vi "Write data.vi"(8 "error in (no error)":errorcluster, 10 "data":T15={"Stop"=FALSE, "dataType"=enum."interferogram", "spectrometerIdx"=0, "buffer size interferogram"=0, "interferogram"={"new"=FALSE, "plot_x_ min"=0.0, "plot_x_max"=0.0, "plot_y_min"=0.0, "plot_y_max"=0.0, "Graph Intrfrgrm"=refnum, "timeStamp"=0, "signal (%)"=0.0, "traces"=[], "traces idx last"=0}, "spectrum"={"new"=FALSE, "plot_x_min"=0.0, "plot_x_max"=0.0, "plot_unit_x"=enum."wavenr/cm", "plot_unit_y"=enum."ADC counts", "plot_y_min"=0.0, "plot_y_max"=0.0, "Graph Spectrum"=refnum, "timeStamp"=0, "X_VAL_OPTIONS"=enum."MIN_MAX", "traces"=[], "traces idx last"=0}, "Thorlabs_OSA_64.lvclass:queue_action.ctlqueue ref"=refnum, "action"=enum."none", "plot zoom step"=0.0, "buffer semaphore"=refnum, "acq stopped"=FALSE, "dataType active"=enum."interferogram", "temperature (degr C)"=0.0, "pressure (hPa)"=0.0, "rel humidity (%)"=0.0, "settings"={"resolution"=0, "sensitivity"=0, "Average"=FALSE, "average nr"=1, "apodisation"=enum."NONE", "acq delay (ms)"=500, "airMesure"=enum."TEMPERATURE", "wmtr on"=FALSE, "intfgrm_smooth_width"=0, "intfgrm_smooth_nrOfPasses"=0, "intfgrm_smooth"=enum."NONE", "phaseCorrection"=enum."NONE", "zeroFill"=0, "spectr_smooth"=enum."NONE", "spectr_smooth_width"=0, "spectr_smooth_nrOfPasses"=0, "resolution (/cm)"=0.0, "REF wavelength, (nm)"=0.0, "gain_idx"=0, "gainAuto"=FALSE, "gain_relative"=0.0, "PD sensitivity mode"=enum."cool: better sensitivity/noise floor", "PD senseMode implemented"=FALSE, "SensorTemperature implemented"=FALSE, "SensorPressure implemented"=FALSE, "SensorHumidity implemented"=FALSE}, "peaks position"=[], "peaks width"=[], "peaks height"=[], "peaks max nr"=0, "peaks latest nr"=0, "peaks new"=FALSE, "power"=0.0, "power new"=FALSE, "path"="", "wavelength (WNr)"=0.0, "wavelength new"=FALSE, "buffer size spectrum"=0, "status"="", "VI reference"=refnum, "funcPointer"=0, "libraryPointer"=0, "singleAcquisition"=FALSE, "coherenceLength (cm)"=0.0, "coherenceLength new"=FALSE, "spectrometer model"="", "spectrometer serial nr"="", "peaks thld left"=[], "peaks thld right"=[], "coherenceLength error (cm)"=0.0, "ADC bits"=0, "peaks position centroid"=[], "peaks height centroid"=[], "OSA series"=enum."OSA200", "channel index spectrum"=0, "spectrometer rangeLow, (/cm)"=0.0, "spectrometer rangeHigh, (/cm)"=0.0, "channel index interferogram"=0} {"peaks height centroid" format="%.2f"; "peaks position centroid" format="%.2f"; "coherenceLength error (cm)" format="%.2f"; "peaks thld right" format="%.2f"; "peaks thld left" format="%.2f"; "coherenceLength (cm)" format="%.2f"; "wavelength (WNr)" format="%.2f"; "power" format="%.2f"; "peaks height" format="%.2f"; "peaks width" format="%.2f"; "peaks position" format="%.2f"; "settings"."REF wavelength, (nm)" format="%.2f"; "settings"."resolution (/cm)" format="%.2f"; "settings"."acq delay (ms)" step=200; "settings"."average nr" min=1 max=100 step=1; "settings"."sensitivity" items=["low", "low medium", "high medium", "high"]; "settings"."resolution" items=["low", "high"]; "rel humidity (%)" format="%.2f"; "pressure (hPa)" format="%.2f"; "temperature (degr C)" format="%.2f"; "plot zoom step" format="%.2f"; "spectrum"."plot_y_max" format="%.2f"; "spectrum"."plot_y_min" format="%.2f"; "spectrum"."plot_x_max" format="%.2f"; "spectrum"."plot_x_min" format="%.2f"; "interferogram"."plot_y_max" format="%.2f"; "interferogram"."plot_y_min" format="%.2f"; "interferogram"."plot_x_max" format="%.2f"; "interferogram"."plot_x_ min" format="%.2f"}, 11 "OSA_FTS in":refnum<class "OSA_FTS.lvclass">) -> (0 "error out":errorcluster, 3 "OSA_FTS out":refnum<class "OSA_FTS.lvclass">)   [LabVIEW 2010, in "OSA_FTS.lvclass"]
uses:
  OSA_FTS.lvclass
  typeDef/acq_dataType.ctl
  OSA.lvclass
  private/graph_intensity.ctl
  typeDef/spectrum_x_unit.ctl
  typeDef/y_unit.ctl
  typeDef/queue_action.ctl
  misc_examples/action_data.ctl
  typeDef/resolution.ctl
  typeDef/sensitivityMode.ctl
  typeDef/apodisation.ctl
  typeDef/airMeasure.ctl
  _misc/Thorlabs_FTS_misc.llb/interferogram_smoothing.ctl
  OSA20X_misc.lvlib
  typeDef/phaseCorrection.ctl
  _misc/Thorlabs_FTS_misc.llb/PDTemperatureMode.ctl
  typeDef/OSA_series.ctl
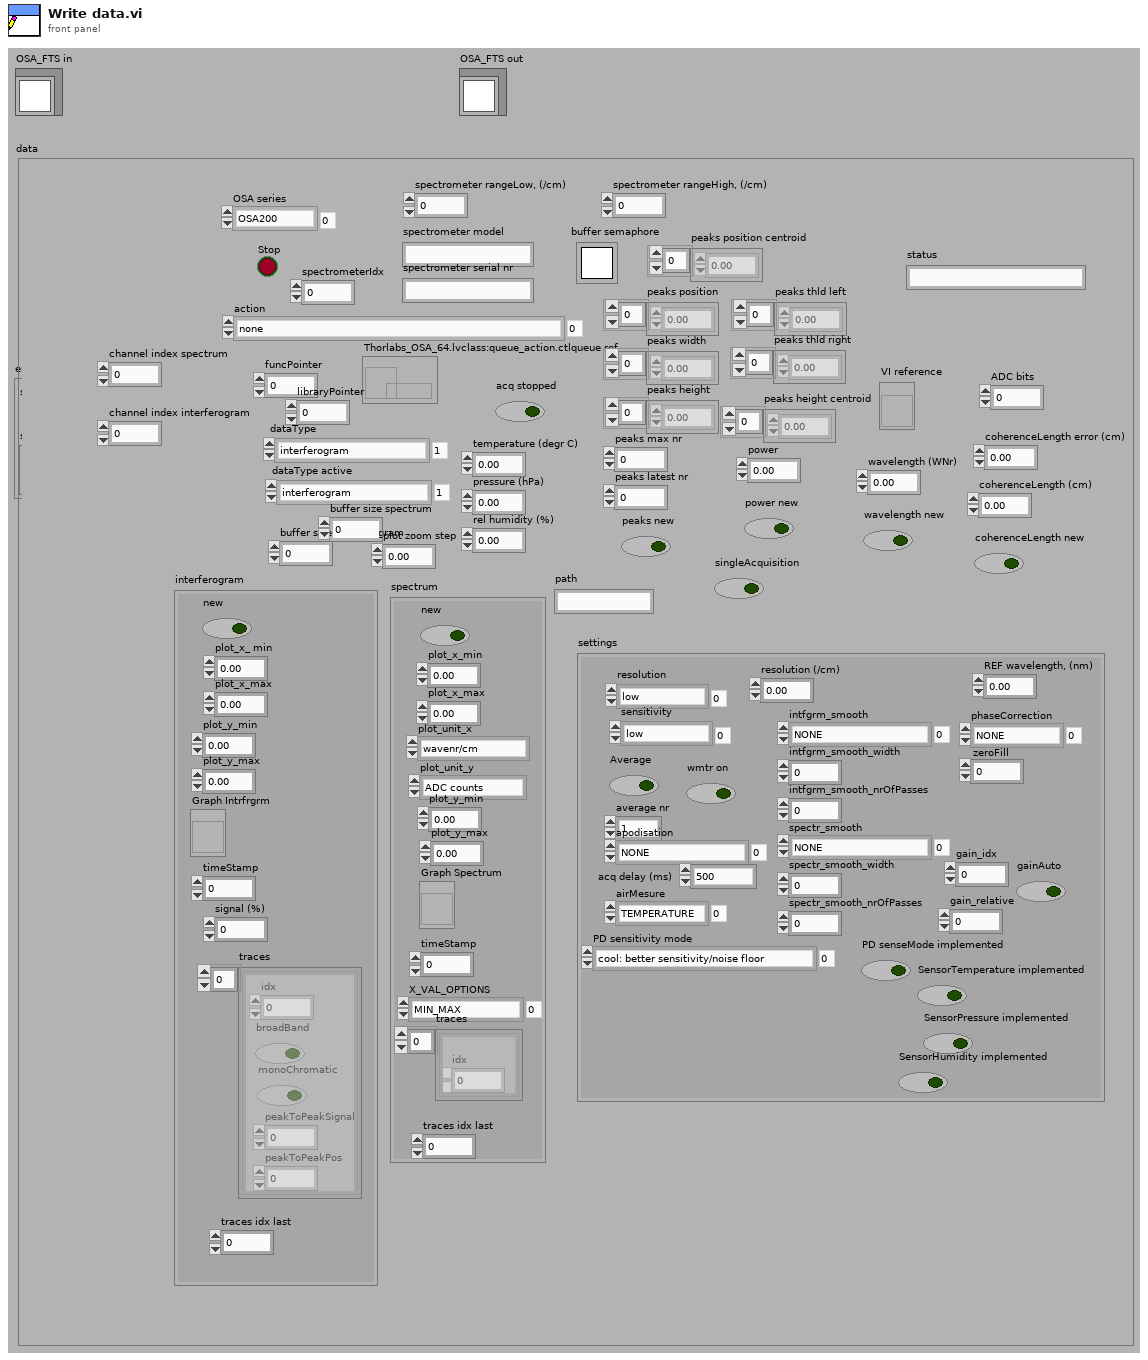
[diagram p1: front panel]
types:
  T1 = typedef "OSA.lvclass/acq_dataType.ctl" = enum16{"none", "interferogram", "spectrum"}
  T2 = typedef "OSA.lvclass/graph_intensity.ctl" = refnum<vi>
  T3 = typedef "OSA.lvclass/spectrum_x_unit.ctl" = enum16{"wavenr/cm", "THz", "eV", "nm_air", "nm_vac"}
  T4 = typedef "OSA.lvclass/y_unit.ctl" = enum16{"ADC counts", "dBm pwr absolute", "dBm pwr density", "mW pwr absolute", "mW pwr density"}
  T5 = typedef "OSA.lvclass/queue_action.ctl" = enum16{"none", "stop", "GUI_plotInterferogram", "GUI_plotSpectrum", "GUI_plotInterferogramRescale", "GUI_plotSpectrumRescale", "GUI_plotInterferogramReset", "GUI_plotSpectrumReset", "GUI_plotInterferogramAutoScaleY", "GUI_plotSpectrumAutoScaleY", "GUI_plotInterferogramZoomOut", "GUI_plotSpectrumZoomOut", "GUI_plotInterferogramPane", "GUI_plotSpectrumPane", "GUI_plotInterferogramZoomMouse", "GUI_plotSpectrumZoomMouse", "GUI_spectrumChannelType", "GUI_channel", "ENVIRONMENT temperature", "ENVIRONMENT pressure", "MODE_resolution set", "MODE_resolution get", "MODE_sensitivity set", "MODE_sensitivity get", "MODE_PDTemperature set", "MODE_PDTemperature get", "REBOOT/RESET firmware", "ACQASYNC_acquireSingleSpectrum", "ACQASYNC_continuous start", "ACQASYNC_continuous stop\n", "ACQASYNC_get last interferogram", "ACQASYNC_get last spectrum", "ACQASYNC_get last waveNr", "ACQOPT_interferogram smoothing set", "ACQOPT_interferogram smoothing get", "ACQOPT_spectrum smoothing set", "ACQOPT_spectrum smoothing get", "ACQOPT_apodisation type set", "ACQOPT_apodisation type get", "ACQOPT_phase correction type set", "ACQOPT_phase correction type get", "ACQOPT_acqIntervall_set", "ACQOPT_acqIntervall_get", "ACQOPT_average spectrum set", "ACQOPT_average spectrum get", "ACQOPT_rolling average set", "ACQOPT_rolling average get", "ACQOPT_zero fill factor set", "ACQOPT_zero fill factor get", "ACQOPT_cycle counting set", "ACQOPT_cycle counting get", "ACQOPT_air measure option set", "ACQOPT_air measure option get", "ACQOPT_gainLevel auto get", "ACQOPT_gainLevel auto set", "ACQOPT_gainLevel get", "ACQOPT_gainLevel set", "ACQOPT_offset set", "ACQOPT_attenuator_auto_set", "ACQOPT_attenuator_set", "ACQOPT_getAll", "INSTRUMENT_PROPERTY_range_WaveNr_min", "INSTRUMENT_PROPERTY_range_WaveNr_max", "INSTRUMENT_PROPERTY_reference_wavelength_cm^-1", "INSTRUMENT_PROPERTY_samplesPerRefPeriod", "INSTRUMENT_PROPERTY_resolution_waveNrPercm", "INSTRUMENT_PROPERTY_availableGainLevels", "INSTRUMENT_PROPERTY_status", "CONVERT", "ANALYSE_POWER", "ANALYSE_PEAKS", "ANALYSE_WAVELENGTH", "ANALYSE_SPECTRUM", "ANALYSE_INTERFEROGRAM", "ANALYSE_COHERENCE_LENGTH", "MATH", "MATH_power", "MATH_peaks", "FILE", "miscellaneous"}
  T6 = typedef "Semaphore RefNum" = refnum<k1>
  T7 = typedef "OSA.lvclass/resolution.ctl" = u16
  T8 = typedef "OSA.lvclass/sensitivityMode.ctl" = u16
  T9 = typedef "OSA.lvclass/apodisation.ctl" = enum16{"NONE", "NORTON_BEER_WEAK", "NORTON_BEER_MEDIUM", "NORTON_BEER_STRONG", "TRIANGULAR", "COSINE", "HANN", "HAMMING", "BLACKMANHARRIS3", "BLACKMANHARRIS4", "GAUSSIAN"}
  T10 = typedef "OSA.lvclass/airMeasure.ctl" = enum16{"TEMPERATURE", "PRESSURE"}
  T11 = typedef "OSA20X_misc.lvlib/interferogram_smoothing.ctl" = enum16{"NONE", "BINOMIAL", "SAVITSKY_GOLAY", "FOURIER", "MOVING_AVERAGE", "GAUSSIAN"}
  T12 = typedef "OSA.lvclass/phaseCorrection.ctl" = enum16{"NONE", "MERTZ", "FORMAN", "MERTZ_FILE", "FORMAN_FILE", "FUTURE COMP."}
  T13 = typedef "OSA20X_misc.lvlib/PDTemperatureMode.ctl" = enum16{"cool: better sensitivity/noise floor", "warm: extended wl range"}
  T14 = typedef "OSA.lvclass/OSA_series.ctl" = enum16{"OSA200", "OSA300", "UNKNOWN"}
  T15 = cluster{"Stop":bool, "dataType":T1, "spectrometerIdx":u16, "buffer size interferogram":i32, "interferogram":cluster{"new":bool, "plot_x_ min":sgl, "plot_x_max":sgl, "plot_y_min":sgl, "plot_y_max":sgl, "Graph Intrfrgrm":T2, "timeStamp":u32, "signal (%)":dbl, "traces":cluster{"idx":u32, "broadBand":bool, "monoChromatic":bool, "peakToPeakSignal":dbl, "peakToPeakPos":dbl}[], "traces idx last":i32}, "spectrum":cluster{"new":bool, "plot_x_min":sgl, "plot_x_max":sgl, "plot_unit_x":T3, "plot_unit_y":T4, "plot_y_min":sgl, "plot_y_max":sgl, "Graph Spectrum":T2, "timeStamp":u32, "X_VAL_OPTIONS":enum16{"MIN_MAX", "ARRAY"}, "traces":cluster{"idx":u32}[], "traces idx last":i32}, "Thorlabs_OSA_64.lvclass:queue_action.ctlqueue ref":refnum<queue>, "action":T5, "plot zoom step":dbl, "buffer semaphore":T6, "acq stopped":bool, "dataType active":T1, "temperature (degr C)":sgl, "pressure (hPa)":sgl, "rel humidity (%)":sgl, "settings":cluster{"resolution":T7, "sensitivity":T8, "Average":bool, "average nr":u32, "apodisation":T9, "acq delay (ms)":u32, "airMesure":T10, "wmtr on":bool, "intfgrm_smooth_width":u16, "intfgrm_smooth_nrOfPasses":u16, "intfgrm_smooth":T11, "phaseCorrection":T12, "zeroFill":u8, "spectr_smooth":T11, "spectr_smooth_width":u16, "spectr_smooth_nrOfPasses":u16, "resolution (/cm)":sgl, "REF wavelength, (nm)":dbl, "gain_idx":u16, "gainAuto":bool, "gain_relative":dbl, "PD sensitivity mode":T13, "PD senseMode implemented":bool, "SensorTemperature implemented":bool, "SensorPressure implemented":bool, "SensorHumidity implemented":bool}, "peaks position":sgl[], "peaks width":sgl[], "peaks height":sgl[], "peaks max nr":u32, "peaks latest nr":i32, "peaks new":bool, "power":dbl, "power new":bool, "path":string, "wavelength (WNr)":dbl, "wavelength new":bool, "buffer size spectrum":i32, "status":string, "VI reference":refnum<vi>, "funcPointer":u64, "libraryPointer":u64, "singleAcquisition":bool, "coherenceLength (cm)":dbl, "coherenceLength new":bool, "spectrometer model":string, "spectrometer serial nr":string, "peaks thld left":sgl[], "peaks thld right":sgl[], "coherenceLength error (cm)":dbl, "ADC bits":u16, "peaks position centroid":sgl[], "peaks height centroid":sgl[], "OSA series":T14, "channel index spectrum":u16, "spectrometer rangeLow, (/cm)":dbl, "spectrometer rangeHigh, (/cm)":dbl, "channel index interferogram":u16}
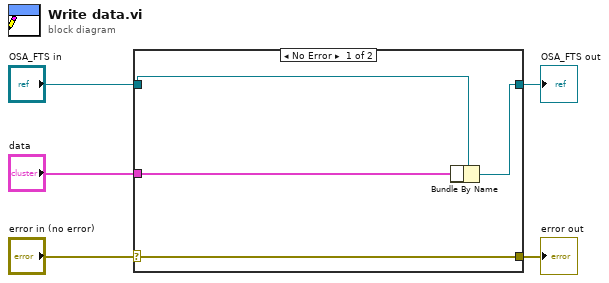
[diagram p0: block diagram]
diagram:
  n1 = case shown="No Error" "error in (no error)" {
    selector: "error in (no error)" -> [w9 w10]
    tunnel: [w9 w10] -> w4
    tunnel: [w7 w11] -> w2
    tunnel: "OSA_FTS in" -> [w8 w11]
    tunnel: "data" -> [w6 _]
    frame No Error {
      n2 = Bundle By Name(cluster=w8, w6) -> (w7:refnum<class "OSA_FTS.lvclass">)
    }
    frame Error {
    }
  }
  "error out" <- w4
  "OSA_FTS out" <- w2
